vi "WriteToCSV_LDO.vi"(6 "StartTime":string, 7 "FVIR?":bool, 10 "PLC Data Out":T1, 11 "file path (dialog if empty)":path) -> ()   [LabVIEW 2020, in "WritingDataFile.lvlib"]
uses:
  WritingDataFile.lvlib
  Modbus/Modbus PLC Data All.ctl
  Modbus/Modbus FVIR Control.ctl
  Modbus/Modbus LDO Control.ctl
  Data to Save.ctl
  <vilib>/Utility/file.llb/Write Delimited Spreadsheet (string).vi
panel:
  out "Data to write to csv":string[](array[string])
  out "file path (dialog if empty) 2":path
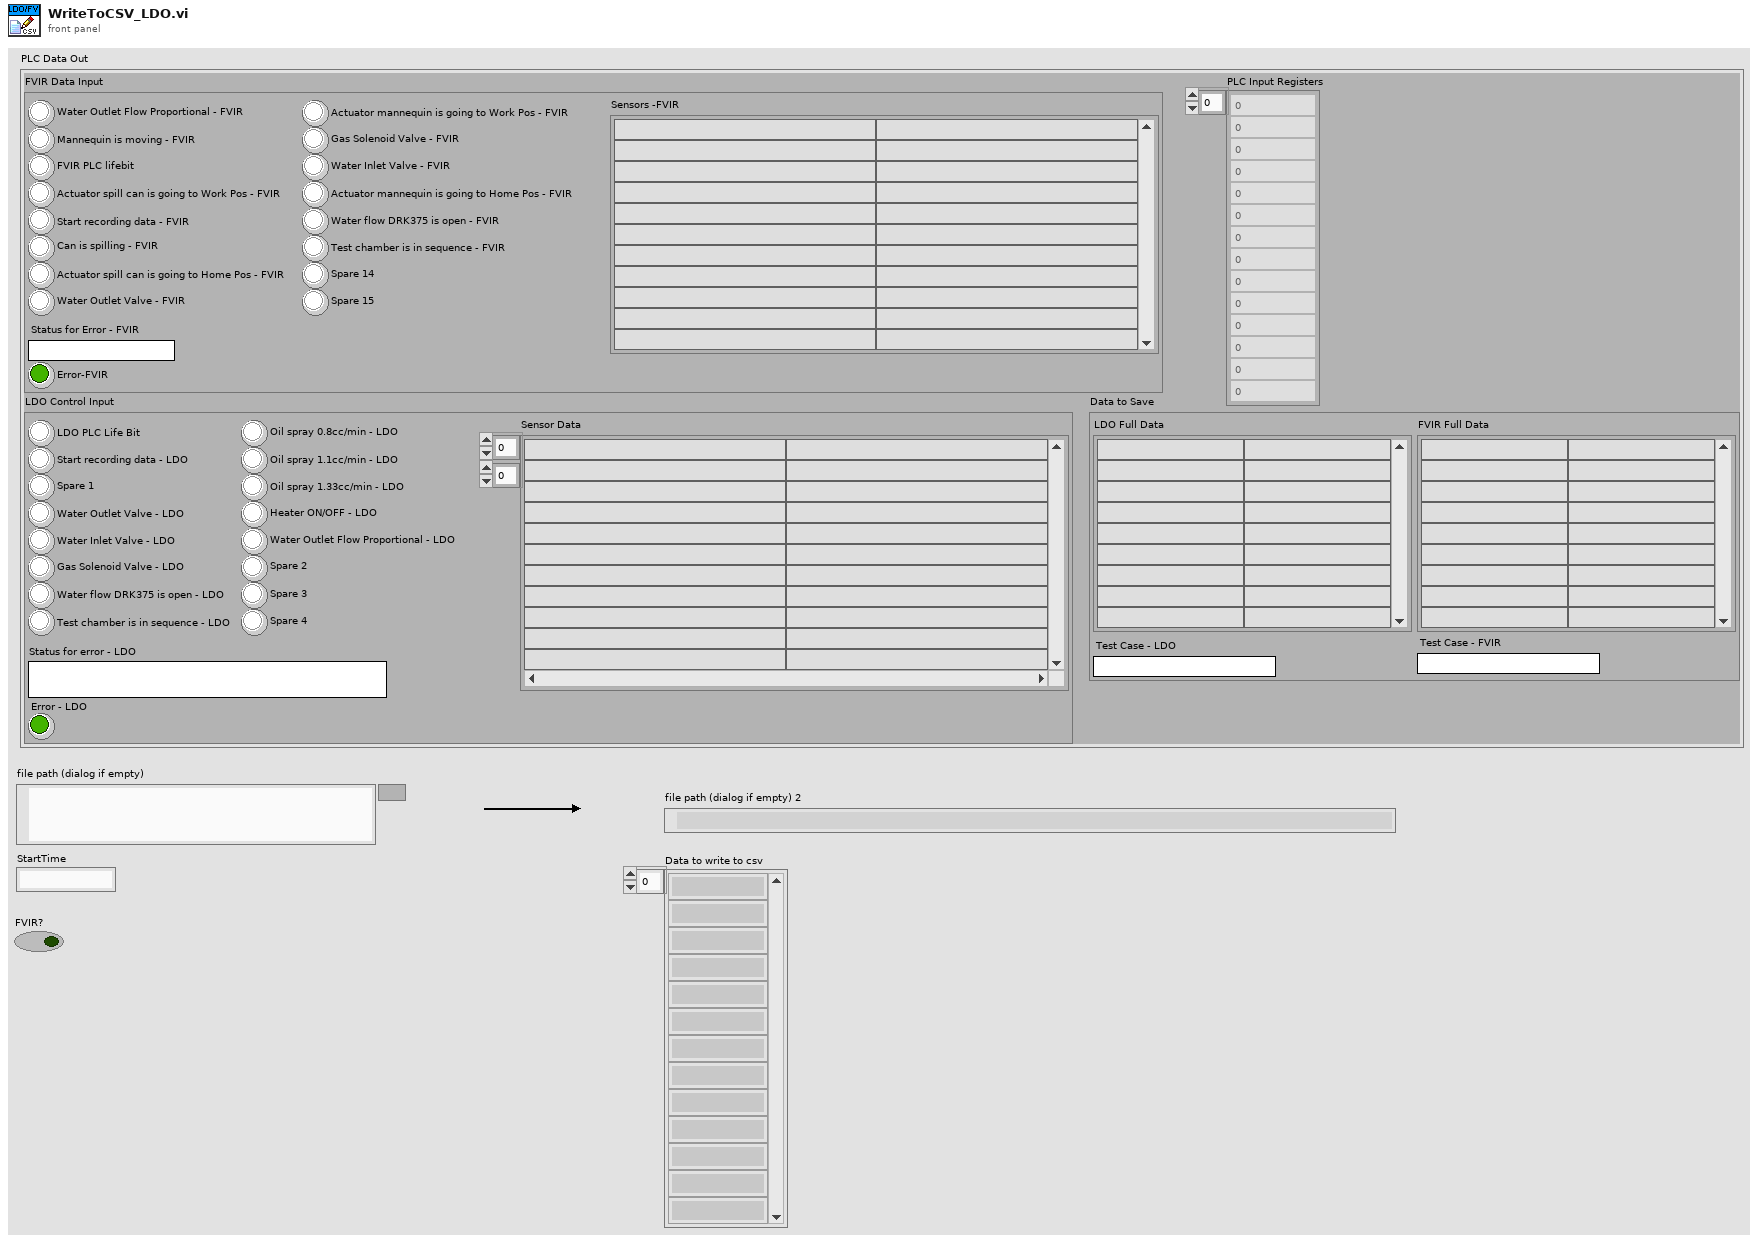
[diagram p1: front panel]
types:
  T1 = typedef "Modbus PLC Data All.ctl" = cluster{"FVIR Data Input":T2, "LDO Control Input":T3, "PLC Input Registers":u16[], "Data to Save":T4}
  T2 = typedef "Modbus FVIR Control.ctl" = cluster{"Spare 15":bool, "Spare 14":bool, "Actuator mannequin is going to Work Pos - FVIR":bool, "Actuator mannequin is going to Home Pos - FVIR":bool, "Test chamber is in sequence - FVIR ":bool, "Water flow DRK375 is open - FVIR":bool, "Gas Solenoid Valve - FVIR":bool, "Water Inlet Valve - FVIR":bool, "Water Outlet Flow Proportional - FVIR":bool, "Start recording data - FVIR":bool, "Actuator spill can is going to Work Pos - FVIR":bool, "Actuator spill can is going to Home Pos - FVIR":bool, "Water Outlet Valve - FVIR":bool, "Can is spilling - FVIR":bool, "Mannequin is moving - FVIR":bool, "FVIR PLC lifebit":bool, "Status for Error - FVIR":string, "Error-FVIR":bool, "Sensors -FVIR":string[][]}
  T3 = typedef "Modbus LDO Control.ctl" = cluster{"LDO PLC Life Bit":bool, "Start recording data - LDO":bool, "Spare 1":bool, "Water Outlet Valve - LDO":bool, "Water Inlet Valve - LDO":bool, "Gas Solenoid Valve - LDO":bool, "Water flow DRK375 is open - LDO":bool, "Test chamber is in sequence - LDO":bool, "Oil spray 0.8cc/min - LDO":bool, "Oil spray 1.1cc/min - LDO":bool, "Oil spray 1.33cc/min - LDO":bool, "Heater ON/OFF - LDO":bool, "Water Outlet Flow Proportional - LDO":bool, "Spare 2":bool, "Spare 3":bool, "Spare 4":bool, "Status for error - LDO":string, "Error - LDO":bool, "Sensor Data":string[][]}
  T4 = typedef "Data to Save.ctl" = cluster{"LDO Full Data":string[][], "FVIR Full Data":string[][], "Test Case - FVIR":string, "Test Case - LDO":string}
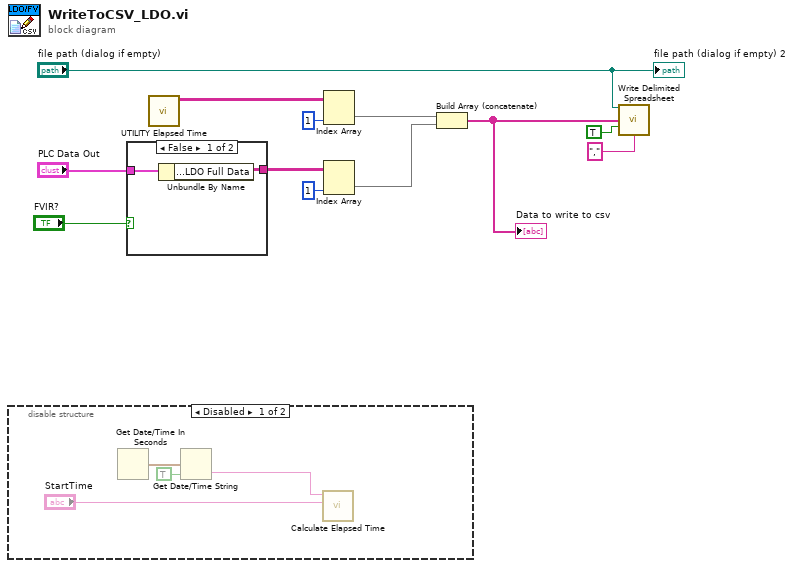
[diagram p0: block diagram]
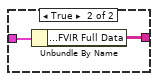
[diagram p3: hidden frame]
diagram:
  n1 = disable-structure shown="Disabled" {
    frame Disabled {
      n2 = Get Date/Time In Seconds() -> (seconds since 1Jan1904=w16:timestamp)
      n3 = Get Date/Time String(seconds (now)=w16, want seconds? (F)=TRUE) -> (time string=w14:string)  [unwired: 1 in, 1 out]
      n4 = call "Calculate Elapsed Time.vi"("StartTime"="StartTime", "time string"=w14) -> ()  [unwired: 9 in, 1 out]
    }
    frame Enabled {
    }
  }
  n5 = case shown="False" "FVIR?" {
    tunnel: "PLC Data Out" -> [w18 w20]
    tunnel: [w17 w19] -> w9
    frame False {
      n6 = Unbundle By Name(w18) -> ("Data to Save.LDO Full Data"=w17:string[][])
    }
    frame True {
      n7 = Unbundle By Name(w20) -> ("Data to Save.FVIR Full Data"=w19:string[][])
    }
  }
  n8 = call "UTILITY Elapsed Time.vi"() -> ("Total Array"=w3:string[][])  [unwired: 7 in, 4 out]
  n9 = Index Array(array=w3, index (col)=1 ("disabled index (col)")) -> (element=w1:string[])  [unwired: 1 in]
  n10 = Index Array(array=w9, index (col)=1 ("disabled index (col)")) -> (element=w7:string[])  [unwired: 1 in]
  n11 = Build Array (concatenate)(w1, w7) -> (w12:string[])
  "Data to write to csv" <- w12
  n12 = call-poly <vilib>:"Write Delimited Spreadsheet.vi"("file path (dialog if empty)"="file path (dialog if empty)", "1D data"=w12, "append to file? (new file:F)"=TRUE, "delimiter (\\t)"="," ("delimiter (\\t)")) -> ()  [unwired: 10 in, 2 out]
  "file path (dialog if empty) 2" <- "file path (dialog if empty)"
